vi "trad ligne chiffre to lettre.vi"(10 "in":string) -> (2 "out":string)   [LabVIEW 2019]
uses:
  <vilib>/regexp/Match Regular Expression.xnode
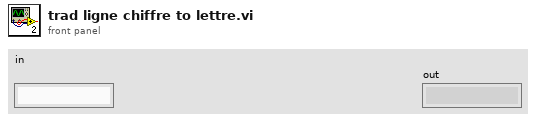
[diagram p1: front panel]
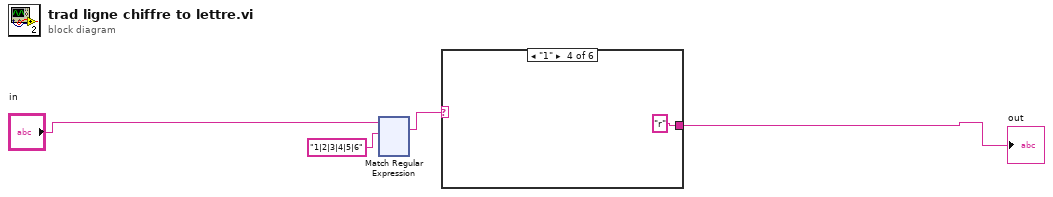
[diagram p0: block diagram]
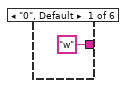
[diagram p2: hidden frame]
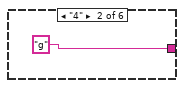
[diagram p3: hidden frame]
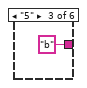
[diagram p4: hidden frame]
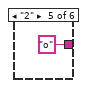
[diagram p5: hidden frame]
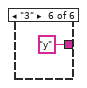
[diagram p6: hidden frame]
diagram:
  n1 = xnode "Match Regular Expression"("input string"="in", "regular expression"="1|2|3|4|5|6" ("input string")) -> ("whole match"=w3:string)  [unwired: 4 in, 4 out]
  n2 = case shown="\"1\"" w3 {
    tunnel: ["w" "g" "b" "r" "o" "y"] -> w2
    frame "0", Default {
    }
    frame "4" {
    }
    frame "5" {
    }
    frame "1" {
    }
    frame "2" {
    }
    frame "3" {
    }
  }
  "out" <- w2
